vi "Get Values To Write.vi"(8 "error in (no error)":errorcluster, 11 "Output Sequencer in":refnum<class "Output Sequencer.lvclass">) -> (0 "error out":errorcluster, 1 "Digital Values to Write":bool[](array[boolean]), 2 "Analog Values to Write":dbl[](array[numeric]), 3 "Output Sequencer out":refnum<class "Output Sequencer.lvclass">, 5 "Sequence State Channels to Write":dbl[](array[numeric]))   [LabVIEW 2020, in "Output Sequencer.lvlib" / "Output Sequencer.lvclass"]
uses:
  Output Sequencer.lvclass
  Output Sequencer.lvclass/Output Sequencer.ctl
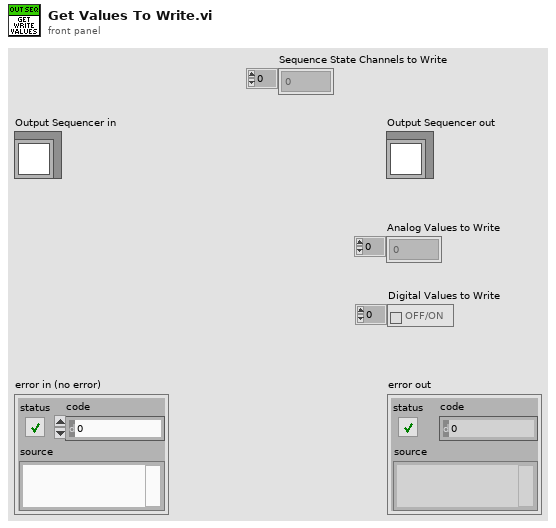
[diagram p1: front panel]
types:
  T1 = typedef "Output Sequencer.lvlib/Output Sequencer.lvclass/Sequencer State.ctl" = enum16{"Error", "Initialize", "Prepare channels", "Wait for test", "Wait for %.1f sec", "Wait for trigger", "Stop condition", "Wait for resume", "Running", "Paused", "No valid step", "Stopped"}
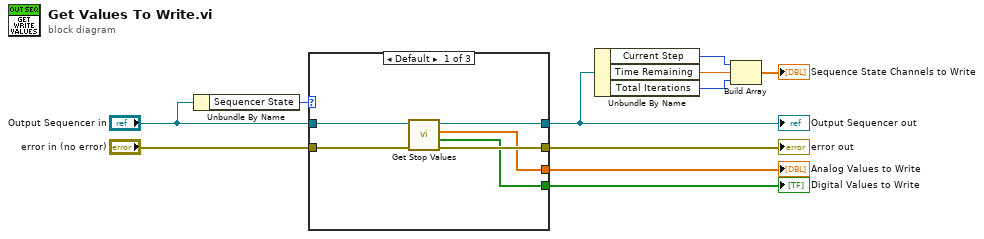
[diagram p0: block diagram]
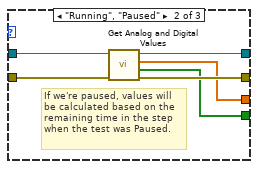
[diagram p2: hidden frame]
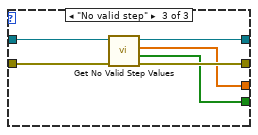
[diagram p3: hidden frame]
diagram:
  n1 = Unbundle By Name("Output Sequencer in") -> ("Sequencer State"=w1:T1)
  n2 = case shown="Default" w1 {
    tunnel: "Output Sequencer in" -> [w17 w23 w26]
    tunnel: "error in (no error)" -> [w16 w22 w29]
    tunnel: [w15 w21 w27] -> w7
    tunnel: [w14 w20 w28] -> w6
    tunnel: [w13 w19 w25] -> w5
    tunnel: [w12 w18 w24] -> w4
    frame Default {
      n3 = call "Get Stop Values.vi"("error in (no error)"=w16, "Output Sequencer in"=w17) -> ("error out"=w14:errorcluster, "Digital Values to Write"=w12:bool[], "Analog Values to Write"=w13:dbl[], "Output Sequencer out"=w15:refnum<class "Output Sequencer.lvclass">)  [unwired: 6 in]
    }
    frame "Running", "Paused" {
      # "If we're paused, values will\nbe calculated based on the\nremaining time in the step\nwhen the test was Paused."
      n4 = call "Get Analog and Digital Values.vi"("error in (no error)"=w22, "Output Sequencer in"=w23) -> ("error out"=w20:errorcluster, "Digital Values to Write"=w18:bool[], "Analog Values to Write"=w19:dbl[], "Output Sequencer out"=w21:refnum<class "Output Sequencer.lvclass">)  [unwired: 6 in]
    }
    frame "No valid step" {
      n5 = call "Get No Valid Step Values.vi"("error in (no error)"=w29, "Output Sequencer in"=w26) -> ("error out"=w28:errorcluster, "Digital Values to Write"=w24:bool[], "Analog Values to Write"=w25:dbl[], "Output Sequencer out"=w27:refnum<class "Output Sequencer.lvclass">)  [unwired: 6 in]
    }
  }
  "Output Sequencer out" <- w7
  "Digital Values to Write" <- w4
  "Analog Values to Write" <- w5
  "error out" <- w6
  n6 = Unbundle By Name(w7) -> ("Current Step"=w8:i32, "Time Remaining"=w10:dbl, "Total Iterations"=w9:i32)
  n7 = Build Array(w8, w10, w9) -> (→"Sequence State Channels to Write":dbl[])
